vi "Day04-03_참조를 통한 객체 관리.vi"() -> ()   [LabVIEW 2021]
panel:
  in  "불리언 3":bool
  in  "불리언 2":bool
  in  "불리언":bool
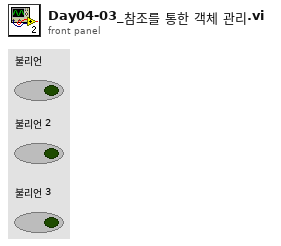
[diagram p1: front panel]
types:
  T1 = enum8{"Enabled", "Disabled", "Disabled and Grayed Out"}
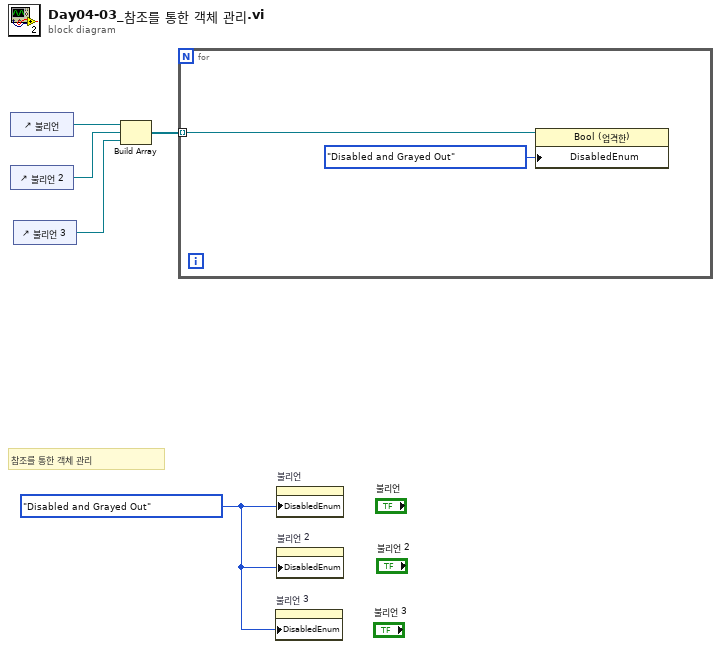
[diagram p0: block diagram]
diagram:
  w2 = T1."Disabled and Grayed Out" ("비활성화")
  # "참조를 통한 객체 관리"
  n1 = control-ref of="불리언"() -> (w5:refnum<vi>)
  n2 = control-ref of="불리언 2"() -> (w4:refnum<vi>)
  n3 = control-ref of="불리언 3"() -> (w1:refnum<vi>)
  n4 = Build Array(w5, w4, w1) -> (w3:refnum<vi>[])
  n5 = for {
    tunnel: w3 -> [w7] mode=indexing
    n6 = property class="Bool (엄격한)"(reference=w7, "DisabledEnum"=T1."Disabled and Grayed Out" ("비활성화")) -> ()  [unwired: 1 in, 2 out]
  }
  n7 = property on="불리언 3" class="Bool (엄격한)"("DisabledEnum"=w2) -> ()  [unwired: 2 in, 2 out]
  n8 = property on="불리언" class="Bool (엄격한)"("DisabledEnum"=w2) -> ()  [unwired: 2 in, 2 out]
  n9 = property on="불리언 2" class="Bool (엄격한)"("DisabledEnum"=w2) -> ()  [unwired: 2 in, 2 out]
